vi "Write TcpClient.vi"(8 "error in (no error)":errorcluster, 10 "TcpClient":refnum<k24>, 11 "dotNET TCP Socket in":refnum<class "dotNET TCP Socket.lvclass">) -> (0 "error out":errorcluster, 3 "dotNET TCP Socket out":refnum<class "dotNET TCP Socket.lvclass">)   [LabVIEW 2013, in "dotNET SSL Socket.lvlib" / "dotNET TCP Socket.lvclass"]
uses:
  dotNET TCP Socket.lvclass
  dotNET TCP Socket.lvclass/dotNET TCP Socket.ctl
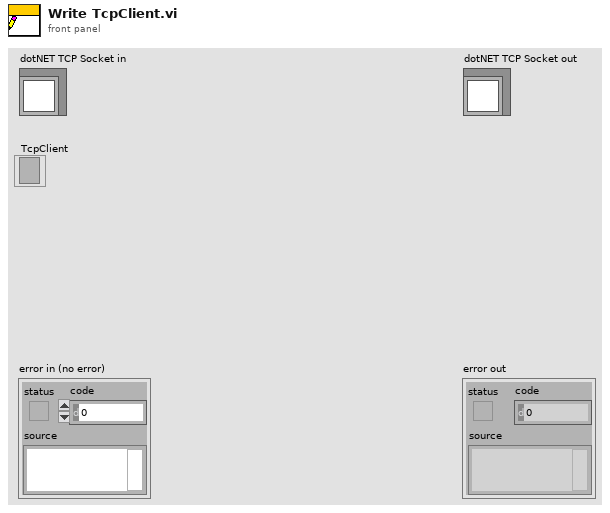
[diagram p1: front panel]
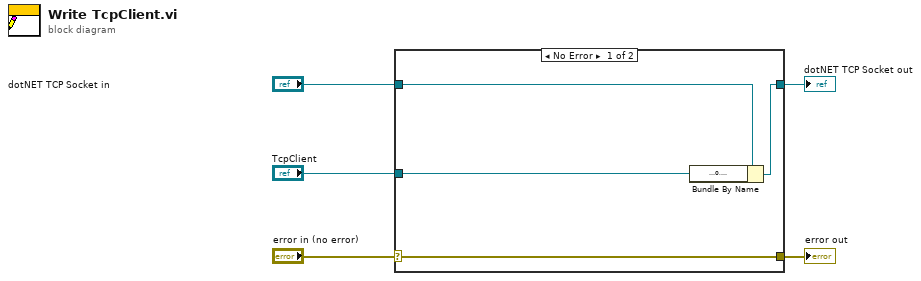
[diagram p0: block diagram]
diagram:
  n1 = case shown="No Error" "error in (no error)" {
    selector: "error in (no error)" -> [w9 w10]
    tunnel: [w9 w10] -> w4
    tunnel: [w7 w11] -> w2
    tunnel: "dotNET TCP Socket in" -> [w8 w11]
    tunnel: "TcpClient" -> [w6 _]
    frame No Error {
      n2 = Bundle By Name(cluster=w8, "TcpClient"=w6) -> (w7:refnum<class "dotNET TCP Socket.lvclass">)
    }
    frame Error {
    }
  }
  "error out" <- w4
  "dotNET TCP Socket out" <- w2
